vi "test simulation.vi"() -> ()   [LabVIEW 2017]
panel:
  in  "IsActive?":bool
  out "Ack":string[](array[string])
  out "Trig":string[](array[string])
  in  "stop":bool
  in  "cid":i32 min=0 max=101 step=1
  in  "Input Status":bool[][](array[boolean])
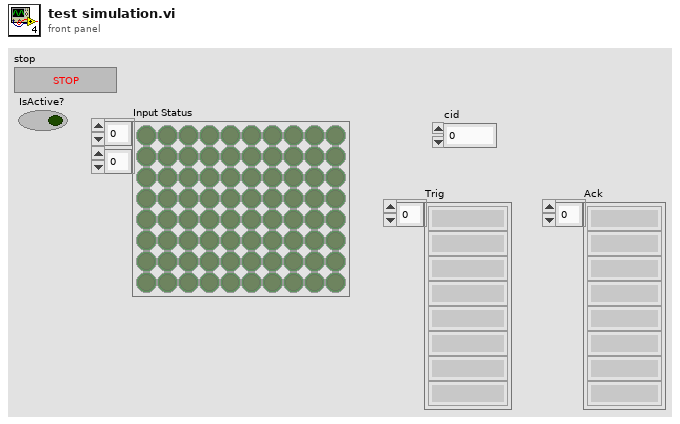
[diagram p1: front panel]
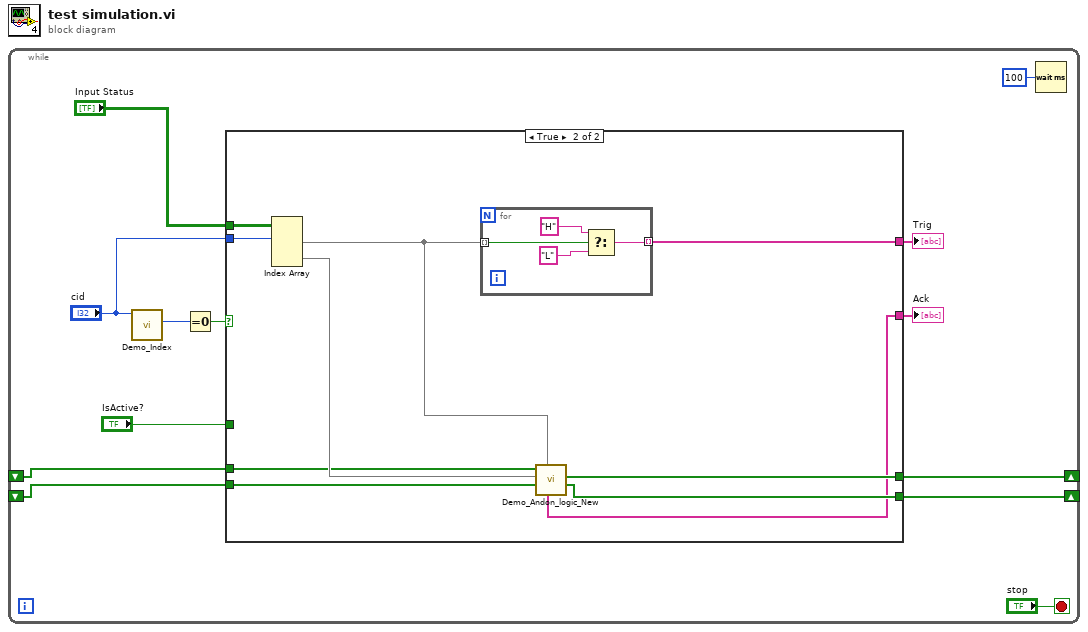
[diagram p0: block diagram]
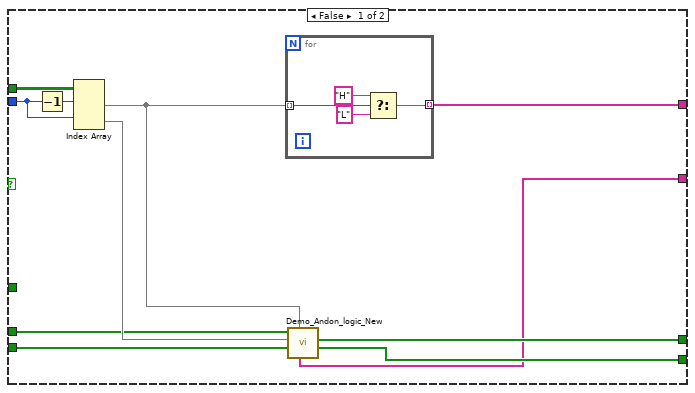
[diagram p2: hidden frame]
diagram:
  n1 = while {
    shift-right: [w5] -> _
    shift-left: _ -> [w4]
    shift-right: [w3] -> _
    shift-left: _ -> [w2]
    stop <- "stop" stop-if-true
    n2 = call "Demo_Index.vi"("Index IN"="cid") -> ("Trig0/Ack1"=w10:i32)  [unwired: 9 in, 1 out]
    n3 = Equal To 0?(x=w10) -> (x = 0?=w11:bool)
    n4 = case shown="True" w11 {
      tunnel: "Input Status" -> [w24 w38]
      tunnel: "cid" -> [w23 w37]
      tunnel: [w21 w36] -> w7
      tunnel: [w15 w29] -> w6
      tunnel: [w19 w32] -> w5
      tunnel: w4 -> [w18 w33]
      tunnel: [w17 w30] -> w3
      tunnel: w2 -> [w16 w31]
      tunnel: "IsActive?" -> [_ _]
      frame False {
        n5 = Decrement(x=w23) -> (x-1=w22:i32)
        n6 = Index Array(array=w24, index (row) #1=w22, index (row) #2=w23) -> (element #1=w14:bool[], element #2=w20:bool[])  [unwired: 2 in]
        n7 = for {
          tunnel: w14 -> [w27] mode=indexing
          tunnel: [w28] -> w21 mode=indexing
          n8 = Select(t="H", s=w27, f="L") -> (s? t:f=w28:string)
        }
        n9 = call "Demo_Andon_logic_New.vi"("Trigger"=w14, "Inputs past"=w16, "Inputs"=w20, "Outputs past"=w18) -> ("Inputs to save"=w17:bool[], "Outputs OUT"=w19:bool[], "Outputs to card"=w15:string[])  [unwired: 5 in]
      }
      frame True {
        n10 = Index Array(array=w38, index (row) #1=w37) -> (element #1=w34:bool[], element #2=w35:bool[])  [unwired: 3 in]
        n11 = for {
          tunnel: w34 -> [w41] mode=indexing
          tunnel: [w40] -> w36 mode=indexing
          n12 = Select(t="H", s=w41, f="L") -> (s? t:f=w40:string)
        }
        n13 = call "Demo_Andon_logic_New.vi"("Trigger"=w34, "Inputs past"=w31, "Inputs"=w35, "Outputs past"=w33) -> ("Inputs to save"=w30:bool[], "Outputs OUT"=w32:bool[], "Outputs to card"=w29:string[])  [unwired: 5 in]
      }
    }
    "Trig" <- w7
    "Ack" <- w6
    n14 = Wait (ms)(milliseconds to wait=u32 100) -> ()  [unwired: 1 out]
  }
